vi "Circle.vi"() -> ()   [LabVIEW 2018]
panel:
  out "Area":dbl
  out "Circumferrence":dbl
  out "Diameter":dbl
  in  "Radius":dbl
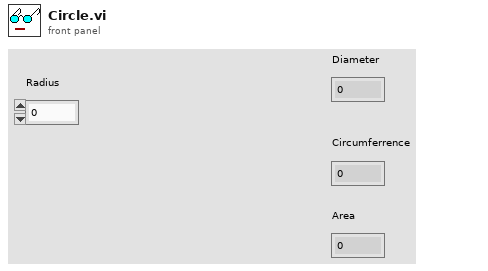
[diagram p1: front panel]
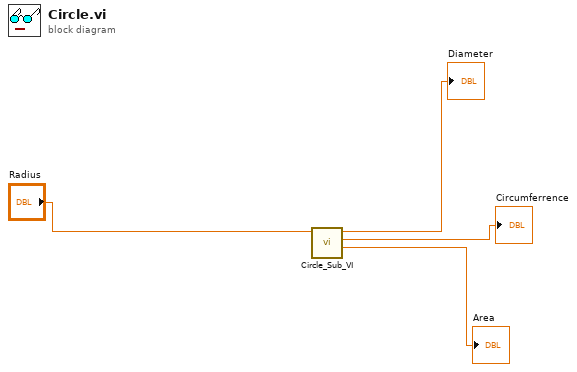
[diagram p0: block diagram]
diagram:
  n1 = call "Circle_Sub_VI.vi"("Radius"="Radius") -> ("Area"=→"Area":dbl, "Circumferrence"=→"Circumferrence":dbl, "Diameter"=→"Diameter":dbl)  [unwired: 8 in]
